vi "Check Leap Year Day.vi"(5 "time":T1) -> (2 "day":u16)   [LabVIEW 2020]
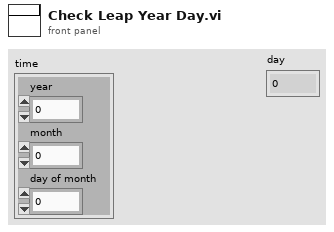
[diagram p1: front panel]
types:
  T1 = cluster{"year":u16, "month":u16, "day of month":u16}
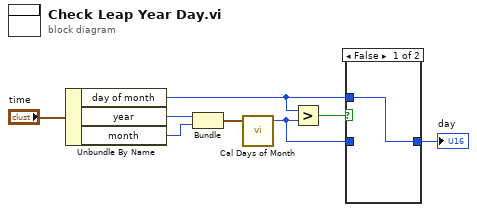
[diagram p0: block diagram]
diagram:
  n1 = Unbundle By Name("time") -> ("day of month"=w3:u16, "year"=w7:u16, "month"=w6:u16)
  n2 = Bundle("year"=w7, "month"=w6) -> (w5:cluster{"year":u16, "month":u16})  [unwired: 1 in]
  n3 = call "Cal Days of Month.vi"("date"=w5) -> ("days"=w2:u16)  [unwired: 4 in]
  n4 = Greater?(x=w3, y=w2) -> (0:w4:bool)
  n5 = case shown="False" w4 {
    tunnel: w3 -> [w9 _]
    tunnel: w2 -> [_ w10]
    tunnel: [w9 w10] -> w1
    frame False {
    }
    frame True {
    }
  }
  "day" <- w1
